vi "TLC Main.vi"(8 "error in (no error)":errorcluster) -> (0 "error out":errorcluster)   [LabVIEW 2018]
doc: "This is the main user interface for the Theatre Light Control Software."
uses:
  Controls/tlc_Cue_Information.ctl
  Controls/channel.ctl
  Controls/tlc_Consumer Control.ctl
  Controls/tlc_Functions.ctl
  Controls/tlc_User Interface Command.ctl
  Controls/tlc_User Interface Data Type.ctl
  Modules/Error/tlc_Error Module Command Control.ctl
  Controls/Play Structure Names.ctl
  Modules/Cue/tlc_Cue_Information Command.ctl
  Modules/File/tlc_File_Command Control.ctl
  Modules/Timing/tlc_Timing Stop Module Control.ctl
  Instance          14 16Saved   TLC Main .vi
  Instance          15 16Saved   TLC Main .vi
panel:
  out "Cue Information":T1 {"Channels"."Intensity" min=0.0 max=100.0 step=1.0 format="%#.0f"}
  in  "Delete":bool
  in  "Down":bool
  in  "Up":bool
  in  "Stop":bool
  in  "Record":bool
  in  "Play":bool
  in  "Cue List":i32(listbox)
  # "Cue Control"
  # "Cue Information"
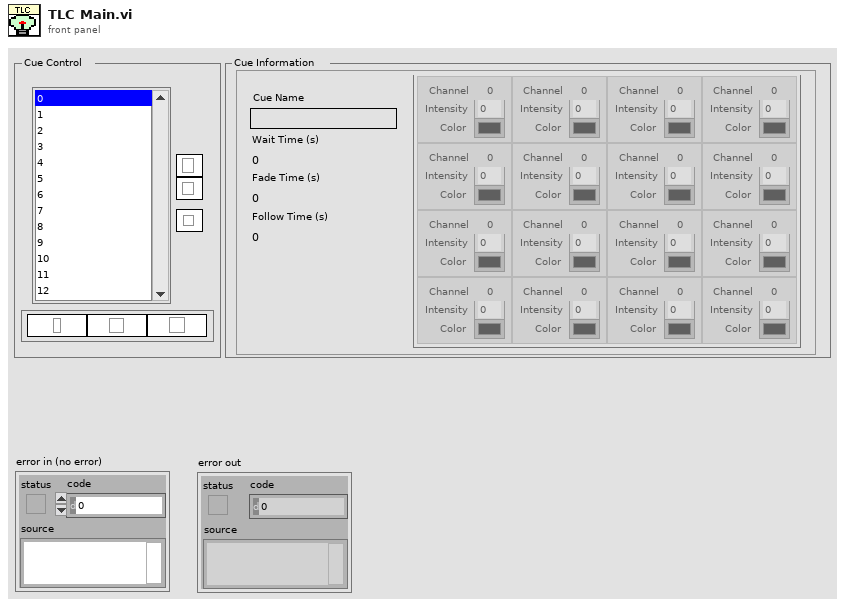
[diagram p1: front panel]
types:
  T1 = typedef "tlc_Cue_Information.ctl" = cluster{"Cue Name":string, "Wait Time (s)":u32, "Fade Time (s)":u32, "Follow Time (s)":u32, "Channels":T2[][]}
  T2 = typedef "channel.ctl" = cluster{"Intensity":dbl, " Color":u32, "Channel":i32}
  T3 = typedef "tlc_Error Module Command Control.ctl" = enum16{"Initialize", "Handle Errors", "Report Errors"}
  T4 = typedef "tlc_User Interface Command.ctl" = cluster{"Data Type":T5, "Data":variant}
  T5 = typedef "tlc_User Interface Data Type.ctl" = enum16{"Initialize", "Initialize Front Panel", "Update Front Panel Channels", "Select Cue in Cue List", "Enable/Disable Front Panel Controls", "Update Cue List", "Stop"}
  T6 = typedef "tlc_Consumer Control.ctl" = cluster{"Command":T7, "Data":variant}
  T7 = typedef "tlc_Functions.ctl" = enum16{"Initialize", "Record", "Load", "Save", "Play", "Move Cue Up", "Move Cue Down", "Select Cue", "Delete", "Stop", "Exit"}
  T8 = typedef "tlc_Timing Stop Module Control.ctl" = enum16{"Intialize", "Stop"}
  T9 = typedef "tlc_Cue_Information Command.ctl" = enum16{"Add Cue", "Delete Cue", "Get Cue Values", "Set Cue Values", "Swap", "Get Number of Cues", "Initialize", "Get Empty Cue"}
  T10 = typedef "Play Structure Names.ctl" = cluster{"Wait":string, "Fade":string, "Follow":string}
  T11 = typedef "tlc_File_Command Control.ctl" = enum16{"Initialize", "Save Cues", "Load Cues", "Shutdown"}
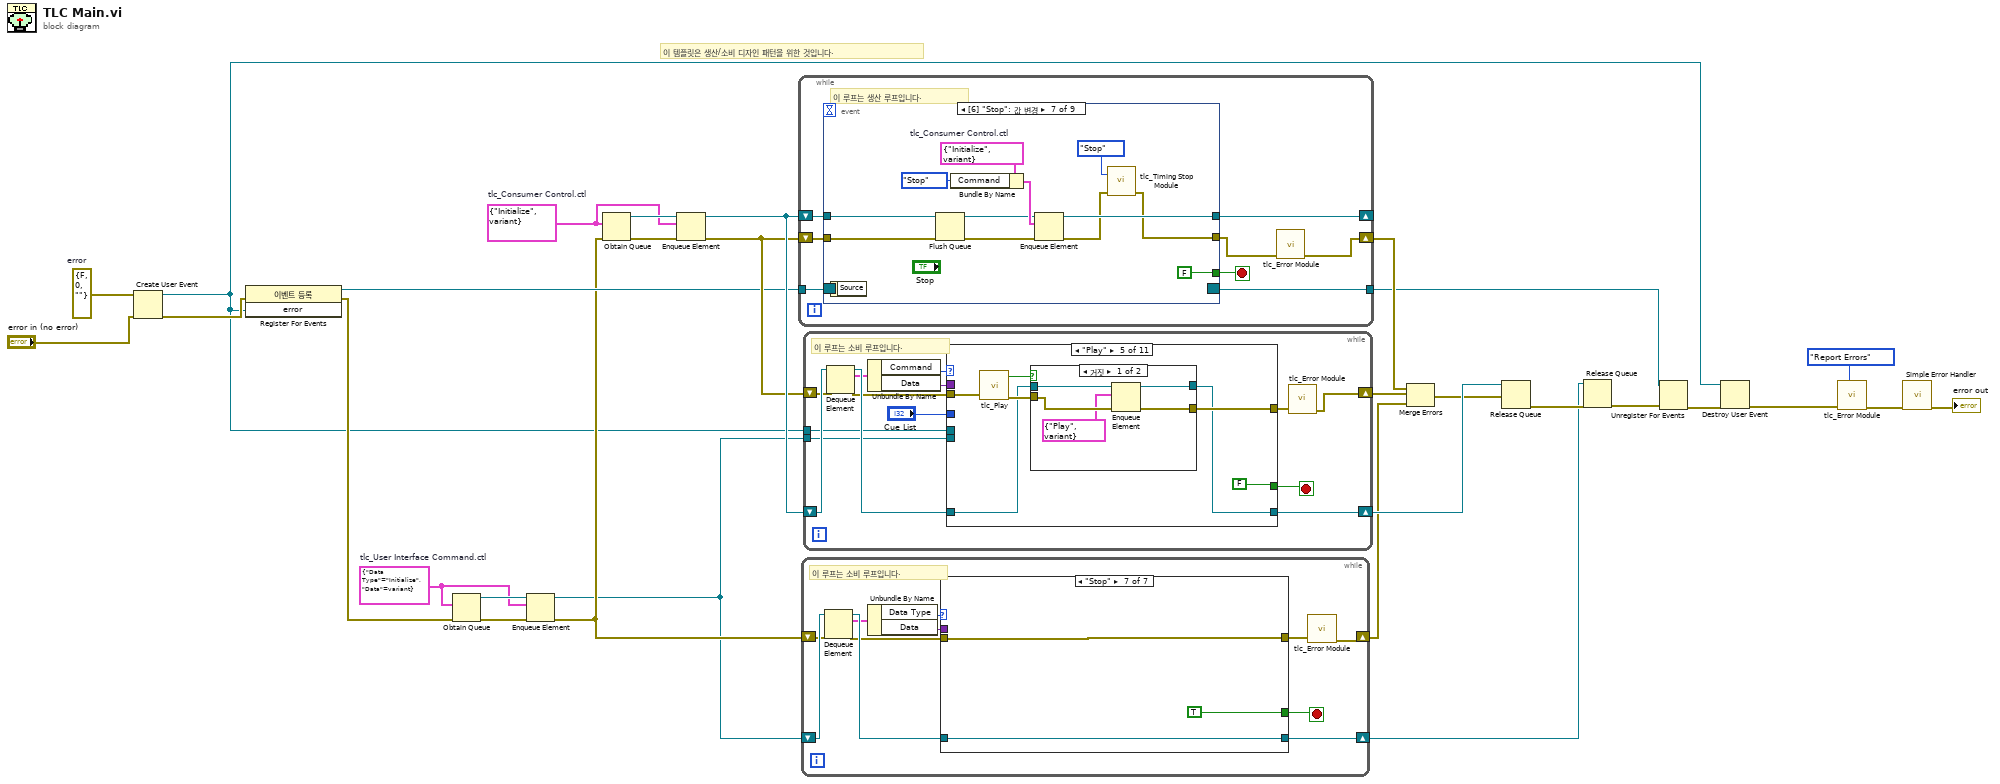
[diagram p0: block diagram]
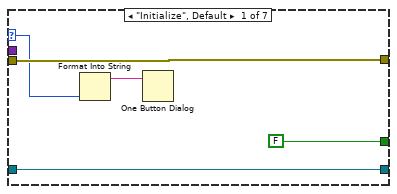
[diagram p2: hidden frame]
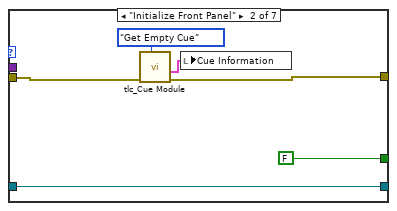
[diagram p3: hidden frame]
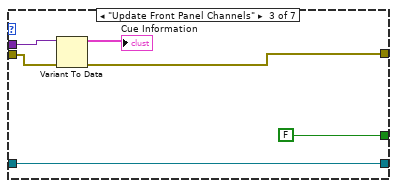
[diagram p4: hidden frame]
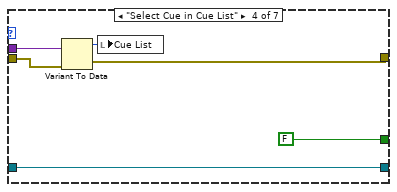
[diagram p5: hidden frame]
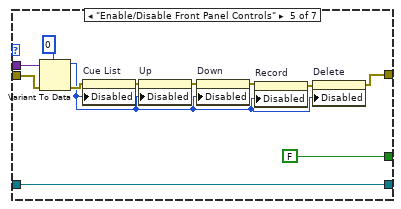
[diagram p6: hidden frame]
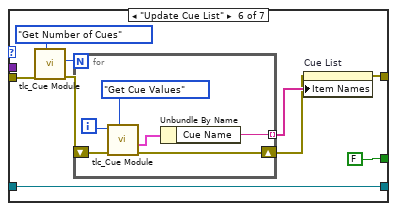
[diagram p7: hidden frame]
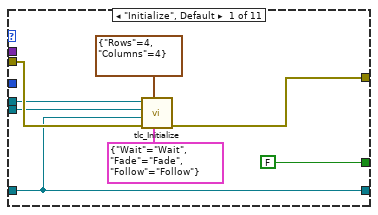
[diagram p8: hidden frame]
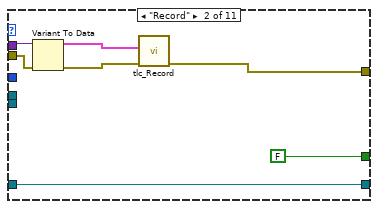
[diagram p9: hidden frame]
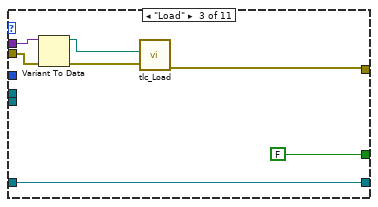
[diagram p10: hidden frame]
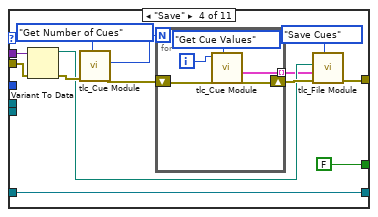
[diagram p11: hidden frame]
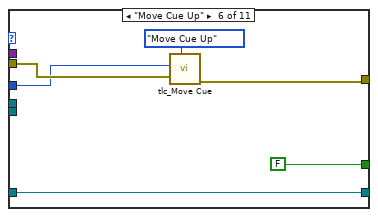
[diagram p13: hidden frame]
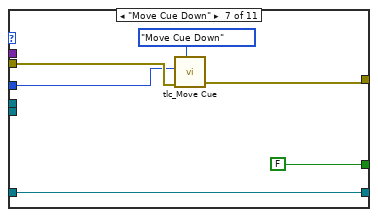
[diagram p14: hidden frame]
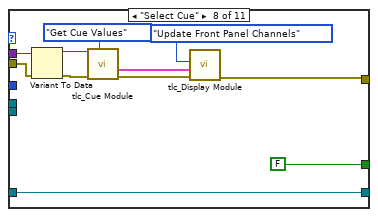
[diagram p15: hidden frame]
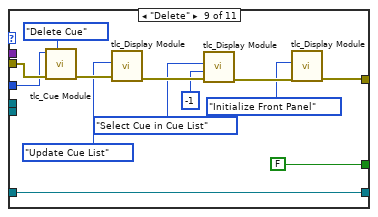
[diagram p16: hidden frame]
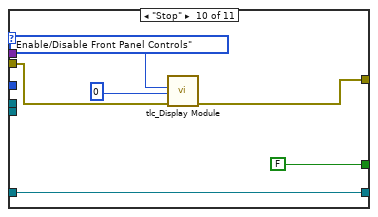
[diagram p17: hidden frame]
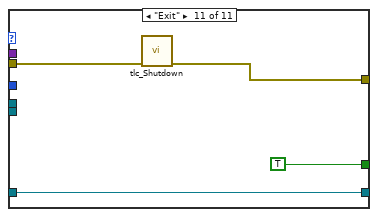
[diagram p18: hidden frame]
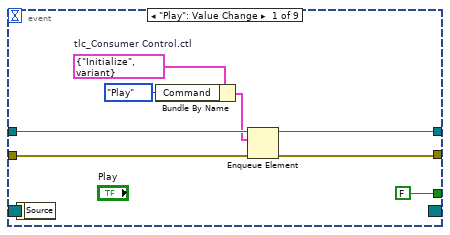
[diagram p19: hidden frame]
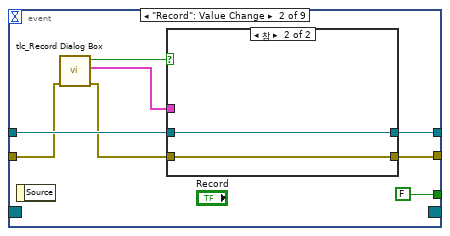
[diagram p20: hidden frame]
diagram:
  w13 = T4 {"Data Type"=enum."Initialize", "Data"=variant}  # tlc_User Interface Command.ctl
  w25 = errorcluster {"status"=FALSE, "code"=0, "source"=""}  # error
  w27 = T6 {"Command"=enum."Initialize", "Data"=variant}  # tlc_Consumer Control.ctl
  # "이 템플릿은 생산/소비 디자인 패턴을 위한 것입니다."
  n1 = Create User Event(user event datatype=w25, error in="error in (no error)") -> (user event=w7:refnum<user-event>, error out=w24:errorcluster)
  n2 = register-events(error in=w24, w7) -> (reference out=w23:refnum<event-registration>, error out=w12:errorcluster)  [unwired: 1 in]
  n3 = Obtain Queue(element data type=w13, error in (no error)=w12) -> (queue out=w15:refnum<queue>, error out=w14:errorcluster)  [unwired: 3 in, 1 out]
  n4 = Enqueue Element(queue=w15, element=w13, error in (no error)=w14) -> (queue out=w6:refnum<queue>, error out=w11:errorcluster)  [unwired: 1 in, 1 out]
  n5 = Obtain Queue(element data type=w27, error in (no error)=w11) -> (queue out=w30:refnum<queue>, error out=w29:errorcluster)  [unwired: 3 in, 1 out]
  n6 = Enqueue Element(queue=w30, element=w27, error in (no error)=w29) -> (queue out=w28:refnum<queue>, error out=w26:errorcluster)  [unwired: 1 in, 1 out]
  n7 = while {
    shift-right: [w31] -> w20
    shift-left: w26 -> [w37]
    shift-right: [w35] -> _
    shift-left: w28 -> [w38]
    tunnel: w23 -> [w34]
    tunnel: [w33] -> w17
    stop <- w36 stop-if-true
    # "이 루프는 생산 루프입니다."
    n8 = event shown="[6] \"Stop\": 값 변경" {
      selector: w34 -> [_ _ _ _ _ _ _ _ _]
      dyn-events: [_ _ _ _ _ _ _ _ _] -> w33
      timeout: _ -> [_ _ _ _ _ _ _ _ _]
      tunnel: w38 -> [w45 w53 w71 w79 w88 w96 w108 w114 w164]
      tunnel: w37 -> [w44 w48 w70 w78 w87 w95 w101 w113 w163]
      tunnel: [w43 w52 w69 w77 w86 w94 w98 w111 w163] -> w32
      tunnel: [FALSE FALSE FALSE FALSE FALSE FALSE FALSE w110 w165] -> w36
      tunnel: [w39 w51 w65 w73 w82 w90 w100 w112 w164] -> w35
      event "Play": Value Change {
        w42 = T6 {"Command"=enum."Initialize", "Data"=variant}  # tlc_Consumer Control.ctl
        n9 = event-data() -> ()  [unwired: 1 in, 1 out]
        n10 = Bundle By Name(cluster=w42, "Command"=tlc_Functions."Play") -> (w41:T6)
        n11 = Enqueue Element(queue=w45, element=w41, error in (no error)=w44) -> (queue out=w39:refnum<queue>, error out=w43:errorcluster)  [unwired: 1 in, 1 out]
      }
      event "Record": Value Change {
        n12 = event-data() -> ()  [unwired: 1 in, 1 out]
        n13 = call "tlc_Record Dialog Box.vi"("error in (no error)"=w48) -> ("error out"=w47:errorcluster, "Output Cue"=w49:T1, "Cancelled?"=w50:bool)  [unwired: 8 in]
        n14 = case shown="참" w50 {
          tunnel: w53 -> [w62 w64]
          tunnel: w47 -> [w61 w63]
          tunnel: [w60 w63] -> w52
          tunnel: [w56 w64] -> w51
          tunnel: w49 -> [w55 _]
          frame False {
            w59 = T6 {"Command"=enum."Initialize", "Data"=variant}  # tlc_Consumer Control.ctl
            n15 = Bundle By Name(cluster=w59, "Command"=tlc_Functions."Record", "Data"=w55) -> (w58:T6)
            n16 = Enqueue Element(queue=w62, element=w58, error in (no error)=w61) -> (queue out=w56:refnum<queue>, error out=w60:errorcluster)  [unwired: 1 in, 1 out]
          }
          frame True {
          }
        }
      }
      event "Up": Value Change {
        w68 = T6 {"Command"=enum."Initialize", "Data"=variant}  # tlc_Consumer Control.ctl
        n17 = event-data() -> ()  [unwired: 1 in, 1 out]
        n18 = Bundle By Name(cluster=w68, "Command"=tlc_Functions."Move Cue Up") -> (w67:T6)
        n19 = Enqueue Element(queue=w71, element=w67, error in (no error)=w70) -> (queue out=w65:refnum<queue>, error out=w69:errorcluster)  [unwired: 1 in, 1 out]
      }
      event "Down": Value Change {
        w76 = T6 {"Command"=enum."Initialize", "Data"=variant}  # tlc_Consumer Control.ctl
        n20 = event-data() -> ()  [unwired: 1 in, 1 out]
        n21 = Bundle By Name(cluster=w76, "Command"=tlc_Functions."Move Cue Down") -> (w75:T6)
        n22 = Enqueue Element(queue=w79, element=w75, error in (no error)=w78) -> (queue out=w73:refnum<queue>, error out=w77:errorcluster)  [unwired: 1 in, 1 out]
      }
      event "Cue List": Value Change {
        w85 = T6 {"Command"=enum."Initialize", "Data"=variant}  # tlc_Consumer Control.ctl
        n23 = event-data() -> ("NewVal"=w81:i32)  [unwired: 1 in]
        n24 = Bundle By Name(cluster=w85, "Command"=tlc_Functions."Select Cue", "Data"=w81) -> (w84:T6)
        n25 = Enqueue Element(queue=w88, element=w84, error in (no error)=w87) -> (queue out=w82:refnum<queue>, error out=w86:errorcluster)  [unwired: 1 in, 1 out]
      }
      event "Delete": Value Change {
        w93 = T6 {"Command"=enum."Initialize", "Data"=variant}  # tlc_Consumer Control.ctl
        n26 = event-data() -> ()  [unwired: 1 in, 1 out]
        n27 = Bundle By Name(cluster=w93, "Command"=tlc_Functions."Delete") -> (w92:T6)
        n28 = Enqueue Element(queue=w96, element=w92, error in (no error)=w95) -> (queue out=w90:refnum<queue>, error out=w94:errorcluster)  [unwired: 1 in, 1 out]
      }
      event "Stop": Value Change {
        w107 = T6 {"Command"=enum."Initialize", "Data"=variant}  # tlc_Consumer Control.ctl
        n29 = event-data() -> ()  [unwired: 1 in, 1 out]
        n30 = Flush Queue(queue=w108, error in (no error)=w101) -> (queue out=w104:refnum<queue>, error out=w103:errorcluster)  [unwired: 1 out]
        n31 = Bundle By Name(cluster=w107, "Command"=tlc_Functions."Stop") -> (w106:T6)
        n32 = Enqueue Element(queue=w104, element=w106, error in (no error)=w103) -> (queue out=w100:refnum<queue>, error out=w99:errorcluster)  [unwired: 1 in, 1 out]
        n33 = call "tlc_Timing Stop Module.vi"("Command (Stop)"=tlc_Timing_Stop_Module_Control."Stop", "error in (no error)"=w99) -> ("error out"=w98:errorcluster)  [unwired: 9 in]
      }
      event Menu Selection (User) {
        n34 = event-data() -> ("ItemTag"=w115:string)  [unwired: 1 in]
        n35 = case shown="기본" w115 {
          tunnel: w114 -> [w119 w137 w159 w162]
          tunnel: w113 -> [w118 w136 w157 w161]
          tunnel: [w117 w135 w158 w162] -> w112
          tunnel: [w116 w134 w156 w161] -> w111
          tunnel: [FALSE FALSE TRUE FALSE] -> w110
          frame "Save" {
            n36 = call "File Dialog"() -> ("selected path"=w120:path, "exists"=w122:bool, "cancelled"=w123:bool)  [unwired: 12 in, 1 out]
            n37 = Compound Arithmetic op=OR(w122, invert w123) -> (w121:bool)
            n38 = case shown="참" w121 {
              tunnel: w120 -> [_ w127]
              tunnel: w119 -> [w126 w133]
              tunnel: w118 -> [w125 w132]
              tunnel: [w126 w131] -> w117
              tunnel: [w125 w130] -> w116
              frame False {
              }
              frame True {
                n39 = Bundle By Name(cluster=T6 {"Command"=enum."Save", "Data"=variant} ("element"), "Data"=w127) -> (w128:T6)
                n40 = Enqueue Element(queue=w133, element=w128, error in (no error)=w132) -> (queue out=w131:refnum<queue>, error out=w130:errorcluster)  [unwired: 1 in, 1 out]
              }
            }
          }
          frame "Open" {
            n41 = call "File Dialog2"() -> ("selected path"=w138:path, "exists"=w140:bool, "cancelled"=w141:bool)  [unwired: 12 in, 1 out]
            n42 = Compound Arithmetic op=OR(w140, invert w141) -> (w139:bool)
            n43 = case shown="참" w139 {
              tunnel: w138 -> [_ w145]
              tunnel: w137 -> [w144 w151]
              tunnel: w136 -> [w143 w150]
              tunnel: [w144 w149] -> w135
              tunnel: [w143 w148] -> w134
              frame False {
              }
              frame True {
                n44 = Bundle By Name(cluster=T6 {"Command"=enum."Load", "Data"=variant} ("element"), "Data"=w145) -> (w146:T6)
                n45 = Enqueue Element(queue=w151, element=w146, error in (no error)=w150) -> (queue out=w149:refnum<queue>, error out=w148:errorcluster)  [unwired: 1 in, 1 out]
              }
            }
          }
          frame "Exit" {
            w155 = T6 {"Command"=enum."Initialize", "Data"=variant}  # tlc_Consumer Control.ctl
            n46 = Bundle By Name(cluster=w155, "Command"=tlc_Functions."Exit") -> (w152:T6)
            n47 = Enqueue Element(queue=w159, element=w152, error in (no error)=w157) -> (queue out=w158:refnum<queue>, error out=w156:errorcluster)  [unwired: 1 in, 1 out]
          }
          frame Default {
          }
        }
      }
      event User Event {
        n48 = event-data() -> ("status"=w165:bool)  [unwired: 1 in]
      }
    }
    n49 = call "tlc_Error Module.vi"("error in (no error)"=w32) -> ("error out"=w31:errorcluster)  [unwired: 9 in, 1 out]
  }
  n50 = while {
    shift-right: [w174] -> w9
    shift-left: w6 -> [w176]
    shift-right: [w166] -> w5
    shift-left: w11 -> [w173]
    stop <- w169 stop-if-true
    # "이 루프는 소비 루프입니다."
    n51 = Dequeue Element(queue=w176, error in (no error)=w173) -> (queue out=w175:refnum<queue>, element=w172:T4, error out=w170:errorcluster)  [unwired: 1 in, 1 out]
    n52 = Unbundle By Name(w172) -> ("Data Type"=w171:T5, "Data"=w168:variant)
    n53 = case shown="\"Stop\"" w171 {
      selector: w171 -> [w177 _ _ _ _ _ _]
      tunnel: w175 -> [w181 w187 w193 w199 w211 w220 w228]
      tunnel: [w181 w187 w193 w199 w211 w220 w228] -> w174
      tunnel: w170 -> [w180 w185 w190 w196 w208 w218 w229]
      tunnel: [w180 w184 w188 w194 w201 w214 w229] -> w167
      tunnel: [FALSE FALSE FALSE FALSE FALSE FALSE TRUE] -> w169
      tunnel: w168 -> [_ _ w191 w197 w209 _ _]
      frame "Initialize", Default {
        n54 = Format Into String(w177) -> (resulting string=w178:string)  [unwired: 3 in, 1 out]
        n55 = One Button Dialog(message=w178) -> ()  [unwired: 1 in, 1 out]
      }
      frame "Initialize Front Panel" {
        n56 = call "tlc_Cue Module.vi"("Command"=tlc_Cue_Information_Command."Get Empty Cue", "error in (no error)"=w185) -> ("error out"=w184:errorcluster, "Cue Output"=w182:T1)  [unwired: 6 in, 1 out]
        n57 = local write "Cue Information"(w182) -> ()
      }
      frame "Update Front Panel Channels" {
        n58 = Variant To Data(error in=w190, Variant=w191) -> (data=→"Cue Information":T1, error out=w188:errorcluster)  [unwired: 1 in]
      }
      frame "Select Cue in Cue List" {
        n59 = Variant To Data(error in=w196, Variant=w197) -> (data=w195:i32, error out=w194:errorcluster)  [unwired: 1 in]
        n60 = local write "Cue List"(w195) -> ()
      }
      frame "Enable/Disable Front Panel Controls" {
        n61 = Variant To Data(error in=w208, type=u8 0, Variant=w209) -> (data=w200:u8, error out=w206:errorcluster)
        n62 = property on="Cue List" class="LstBox (엄격한)"(error in=w206, "Disabled"=w200) -> (error out=w205:errorcluster)  [unwired: 1 in, 1 out]
        n63 = property on="Up" class="Bool"(error in=w205, "Disabled"=w200) -> (error out=w204:errorcluster)  [unwired: 1 in, 1 out]
        n64 = property on="Down" class="Bool"(error in=w204, "Disabled"=w200) -> (error out=w203:errorcluster)  [unwired: 1 in, 1 out]
        n65 = property on="Record" class="Bool"(error in=w203, "Disabled"=w200) -> (error out=w202:errorcluster)  [unwired: 1 in, 1 out]
        n66 = property on="Delete" class="Bool"(error in=w202, "Disabled"=w200) -> (error out=w201:errorcluster)  [unwired: 1 in, 1 out]
      }
      frame "Update Cue List" {
        n67 = call "tlc_Cue Module.vi"("Command"=tlc_Cue_Information_Command."Get Number of Cues", "error in (no error)"=w218) -> ("error out"=w215:errorcluster, "Number of Cues"=w216:i32)  [unwired: 6 in, 1 out]
        n68 = for {
          N: w216 -> [_]
          shift-right: [w225] -> w212
          shift-left: w215 -> [w226]
          tunnel: [w221] -> w213 mode=indexing
          i -> [w223]
          n69 = call "tlc_Cue Module.vi"("Command"=tlc_Cue_Information_Command."Get Cue Values", "error in (no error)"=w226, "Cue Index"=w223) -> ("error out"=w225:errorcluster, "Cue Output"=w222:T1)  [unwired: 5 in, 1 out]
          n70 = Unbundle By Name(w222) -> ("Cue Name"=w221:string)
        }
        n71 = property on="Cue List" class="LstBox (엄격한)"(error in=w212, "Item Names"=w213) -> (error out=w214:errorcluster)  [unwired: 1 in, 1 out]
      }
      frame "Stop" {
      }
    }
    n72 = call "tlc_Error Module.vi"("error in (no error)"=w167) -> ("error out"=w166:errorcluster)  [unwired: 9 in, 1 out]
  }
  n73 = while {
    shift-right: [w241] -> w19
    shift-left: w28 -> [w243]
    shift-right: [w231] -> w21
    shift-left: w26 -> [w240]
    tunnel: w7 -> [w234]
    tunnel: w6 -> [w233]
    stop <- w236 stop-if-true
    # "이 루프는 소비 루프입니다."
    n74 = Dequeue Element(queue=w243, error in (no error)=w240) -> (queue out=w242:refnum<queue>, element=w239:T6, error out=w237:errorcluster)  [unwired: 1 in, 1 out]
    n75 = Unbundle By Name(w239) -> ("Command"=w238:T7, "Data"=w235:variant)
    n76 = case shown="\"Play\"" w238 {
      tunnel: w242 -> [w244 w258 w265 w278 w286 w303 w309 w320 w333 w339 w343]
      tunnel: [w244 w258 w265 w278 w284 w303 w309 w320 w333 w339 w343] -> w241
      tunnel: w237 -> [w250 w255 w262 w275 w289 w301 w307 w317 w331 w337 w341]
      tunnel: [w249 w252 w259 w269 w285 w300 w306 w312 w327 w334 w340] -> w232
      tunnel: [FALSE FALSE FALSE FALSE FALSE FALSE FALSE FALSE FALSE FALSE TRUE] -> w236
      tunnel: w235 -> [_ w256 w263 w276 _ _ _ w318 _ _ _]
      tunnel: w234 -> [w246 _ _ _ _ _ _ _ _ _ _]
      tunnel: w233 -> [w245 _ _ _ _ _ _ _ _ _ _]
      tunnel: "Cue List" -> [_ _ _ _ _ w298 w304 _ w326 _ _]
      frame "Initialize", Default {
        n77 = call "tlc_Initialize.vi"("Play Structure Names"=T10 {"Wait"="Wait", "Fade"="Fade", "Follow"="Follow"}, "Number of Channels"=cluster{"Rows":i32, "Columns":i32} {"Rows"=4, "Columns"=4}, "error in (no error)"=w250, "tlc_Consumer Queue Reference.ctl"=w244, "tlc_Display Queue Reference.ctl"=w245, "tlc_User Event Reference.ctl"=w246) -> ("error out"=w249:errorcluster)  [unwired: 5 in]
      }
      frame "Record" {
        n78 = Variant To Data(error in=w255, Variant=w256) -> (data=w253:T1, error out=w254:errorcluster)  [unwired: 1 in]
        n79 = call "tlc_Record.vi"("error in (no error)"=w254, "Cue"=w253) -> ("error out"=w252:errorcluster)  [unwired: 9 in]
      }
      frame "Load" {
        n80 = Variant To Data(error in=w262, Variant=w263) -> (data=w260:path, error out=w261:errorcluster)  [unwired: 1 in]
        n81 = call "tlc_Load.vi"("error in (no error)"=w261, "Path"=w260) -> ("error out"=w259:errorcluster)  [unwired: 9 in]
      }
      frame "Save" {
        n82 = Variant To Data(error in=w275, Variant=w276) -> (data=w268:path, error out=w274:errorcluster)  [unwired: 1 in]
        n83 = call "tlc_Cue Module.vi"("Command"=tlc_Cue_Information_Command."Get Number of Cues", "error in (no error)"=w274) -> ("error out"=w271:errorcluster, "Number of Cues"=w272:i32)  [unwired: 6 in, 1 out]
        n84 = for {
          N: w272 -> [_]
          tunnel: [w280] -> w267 mode=indexing
          shift-right: [w279] -> w270
          shift-left: w271 -> [w283]
          i -> [w281]
          n85 = call "tlc_Cue Module.vi"("Command"=tlc_Cue_Information_Command."Get Cue Values", "error in (no error)"=w283, "Cue Index"=w281) -> ("error out"=w279:errorcluster, "Cue Output"=w280:T1)  [unwired: 5 in, 1 out]
        }
        n86 = call "tlc_File Module.vi"("Command"=tlc_File_Command_Control."Save Cues", "error in (no error)"=w270, "Cue Array Input"=w267, "Path"=w268) -> ("error out"=w269:errorcluster)  [unwired: 6 in, 1 out]
      }
      frame "Play" {
        n87 = call "tlc_Play.vi"("error in (no error)"=w289) -> ("error out"=w287:errorcluster, "Stop?"=w288:bool)  [unwired: 9 in]
        n88 = case shown="거짓" w288 {
          tunnel: w287 -> [w294 w296]
          tunnel: w286 -> [w295 w297]
          tunnel: [w293 w296] -> w285
          tunnel: [w292 w297] -> w284
          frame False {
            n89 = Enqueue Element(queue=w295, element=T6 {"Command"=enum."Play", "Data"=variant}, error in (no error)=w294) -> (queue out=w292:refnum<queue>, error out=w293:errorcluster)  [unwired: 1 in, 1 out]
          }
          frame True {
          }
        }
      }
      frame "Move Cue Up" {
        n90 = call "tlc_Move Cue.vi"("Cue Operation"=enum16{"Move Cue Up", "Move Cue Down"}."Move Cue Up", "error in (no error)"=w301, "Selected Cue"=w298) -> ("error out"=w300:errorcluster)  [unwired: 8 in]
      }
      frame "Move Cue Down" {
        n91 = call "tlc_Move Cue.vi"("Cue Operation"=enum16{"Move Cue Up", "Move Cue Down"}."Move Cue Down", "error in (no error)"=w307, "Selected Cue"=w304) -> ("error out"=w306:errorcluster)  [unwired: 8 in]
      }
      frame "Select Cue" {
        n92 = Variant To Data(error in=w317, Variant=w318) -> (data=w316:i32, error out=w314:errorcluster)  [unwired: 1 in]
        n93 = call "tlc_Cue Module.vi"("Command"=tlc_Cue_Information_Command."Get Cue Values", "error in (no error)"=w314, "Cue Index"=w316) -> ("error out"=w313:errorcluster, "Cue Output"=w311:T1)  [unwired: 5 in, 1 out]
        n94 = call "tlc_Display Module.vi"("error in (no error)"=w313, "Data"=w311, "Data Type"=tlc_User_Interface_Data_Type."Update Front Panel Channels") -> ("error out"=w312:errorcluster)  [unwired: 8 in]
      }
      frame "Delete" {
        n95 = call "tlc_Cue Module.vi"("Command"=tlc_Cue_Information_Command."Delete Cue", "error in (no error)"=w331, "Cue Index"=w326) -> ("error out"=w330:errorcluster)  [unwired: 5 in, 2 out]
        n96 = call "tlc_Display Module.vi"("error in (no error)"=w330, "Data Type"=tlc_User_Interface_Data_Type."Update Cue List") -> ("error out"=w329:errorcluster)  [unwired: 9 in]
        n97 = call "tlc_Display Module.vi"("error in (no error)"=w329, "Data"=-1, "Data Type"=tlc_User_Interface_Data_Type."Select Cue in Cue List") -> ("error out"=w328:errorcluster)  [unwired: 8 in]
        n98 = call "tlc_Display Module.vi"("error in (no error)"=w328, "Data Type"=tlc_User_Interface_Data_Type."Initialize Front Panel") -> ("error out"=w327:errorcluster)  [unwired: 9 in]
      }
      frame "Stop" {
        n99 = call "tlc_Display Module.vi"("error in (no error)"=w337, "Data"=u8 0, "Data Type"=tlc_User_Interface_Data_Type."Enable/Disable Front Panel Controls") -> ("error out"=w334:errorcluster)  [unwired: 8 in]
      }
      frame "Exit" {
        n100 = call "tlc_Shutdown.vi"("error in (no error)"=w341) -> ("error out"=w340:errorcluster)  [unwired: 10 in]
      }
    }
    n101 = call "tlc_Error Module.vi"("error in (no error)"=w232) -> ("error out"=w231:errorcluster)  [unwired: 9 in, 1 out]
  }
  n102 = Merge Errors(w20, w21, w5) -> (w18:errorcluster)
  n103 = Release Queue(queue=w19, error in (no error)=w18) -> (error out=w10:errorcluster)  [unwired: 1 in, 2 out]
  n104 = Release Queue(queue=w9, error in (no error)=w10) -> (error out=w8:errorcluster)  [unwired: 1 in, 2 out]
  n105 = Unregister For Events(event registration refnum=w17, error in=w8) -> (error out=w16:errorcluster)
  n106 = Destroy User Event(user event=w7, error in=w16) -> (error out=w4:errorcluster)
  n107 = call "tlc_Error Module.vi"("Command (Handle Errors"=tlc_Error_Module_Command_Control."Report Errors", "error in (no error)"=w4) -> ("error out"=w3:errorcluster)  [unwired: 8 in, 1 out]
  n108 = call <vilib>:"Simple Error Handler.vi"("error in (no error)"=w3) -> ("error out"=→"error out":errorcluster)  [unwired: 4 in, 4 out]
